vi "IMU Fail Detection.vi"(2 "IMU Value":dbl, 3 "Boolean":bool) -> (0 "Array":string[](array[string]), 1 "IMU Error?":bool)   [LabVIEW 2018]
uses:
  <vilib>/ptbypt/NI_PtbyPt.lvlib
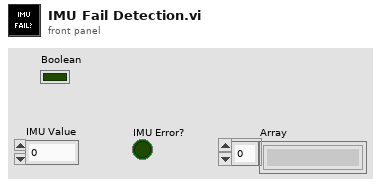
[diagram p1: front panel]
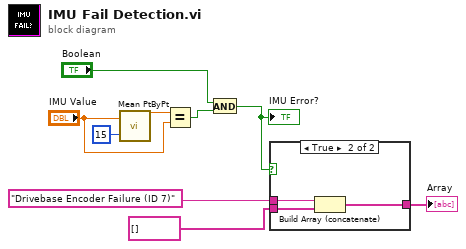
[diagram p0: block diagram]
diagram:
  n1 = call <vilib>:"Mean PtByPt.vi"("x"="IMU Value", "sample length"=15) -> ("mean"=w8:dbl)  [unwired: 2 in, 1 out]
  n2 = Equal?(x=w8, y="IMU Value") -> (x = y?=w2:bool)
  n3 = And(x="Boolean", y=w2) -> (x .and. y?=w1:bool)
  "IMU Error?" <- w1
  n4 = case shown="True" w1 {
    tunnel: string[] [] -> [w10 w13]
    tunnel: "Drivebase Encoder Failure (ID 7)" ("refnum name") -> [_ w12]
    tunnel: [w10 w11] -> w5
    frame False {
    }
    frame True {
      n5 = Build Array (concatenate)(w12, w13) -> (w11:string[])
    }
  }
  "Array" <- w5
